vi "Find Row.vi"(11 "Boarding Pass":string) -> (3 "Row":i32)   [LabVIEW 2020]
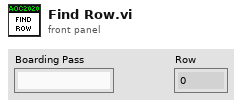
[diagram p1: front panel]
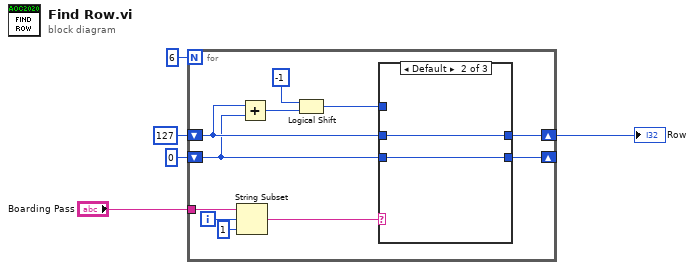
[diagram p0: block diagram]
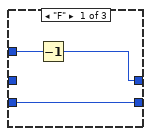
[diagram p2: hidden frame]
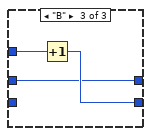
[diagram p3: hidden frame]
diagram:
  n1 = for {
    N: 6 -> [_]
    tunnel: "Boarding Pass" -> [w16]
    shift-right: [w8] -> w2
    shift-left: 127 -> [w7]
    shift-right: [w9] -> _
    shift-left: 0 -> [w6]
    i -> [w15]
    n2 = String Subset(string=w16, offset (0)=w15, length (rest)=1 ("length (rest)")) -> (substring=w11:string)
    n3 = Add(x=w7, y=w6) -> (x+y=w13:i32)
    n4 = Logical Shift(y=i16 -1, x=w13) -> (x << y=w10:i32)
    n5 = case shown="Default" w11 {
      tunnel: w10 -> [w19 _ w24]
      tunnel: [w17 w20 w23] -> w9
      tunnel: [w18 w21 w22] -> w8
      tunnel: w7 -> [_ w21 w22]
      tunnel: w6 -> [w17 w20 _]
      frame "F" {
        n6 = Decrement(x=w19) -> (x-1=w18:i32)
      }
      frame Default {
      }
      frame "B" {
        n7 = Increment(x=w24) -> (x+1=w23:i32)
      }
    }
  }
  "Row" <- w2
